vi "Entrada de datos.vi"(5 "ID":string, 6 "string":string) -> (1 "CAN frame":T1 {"payload" format="%x"; "timestamp" format="%<%.7X\n%x>T"; "type" items=["CAN Data"=0, "CAN Remote"=1, "CAN Bus Error"=2, "CAN 2.0 Data"=8, "CAN FD Data"=16, "CAN FD+BRS Data"=24, "J1939 Data"=192, "Delay"=224, "Log Trigger"=225, "Start Trigger"=226]; "identifier" format="%x"})   [LabVIEW 2022 SP3]
uses:
  <vilib>/xnet/xnet.llb/XNET Frame CAN.ctl
  <vilib>/xnet/xnet.llb/XNET Frame Type CAN.ctl
panel:
  out "unsigned byte array":u8[](array[numeric]) format="%x"
  out "number":u32 format="%x"
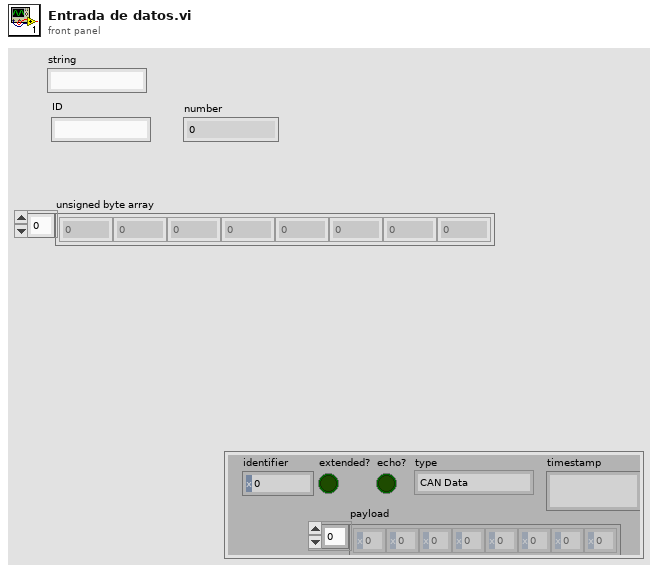
[diagram p1: front panel]
types:
  T1 = typedef "XNET Frame CAN.ctl" = cluster{"timestamp":timestamp, "payload":u8[], "identifier":u32, "type":T2, "extended?":bool, "echo?":bool}
  T2 = typedef "XNET Frame Type CAN.ctl" = u8
  T3 = cluster{"timestamp":timestamp, "unsigned byte array":u8[], u32, "type":T2, "Extended":bool, "Echo":bool}
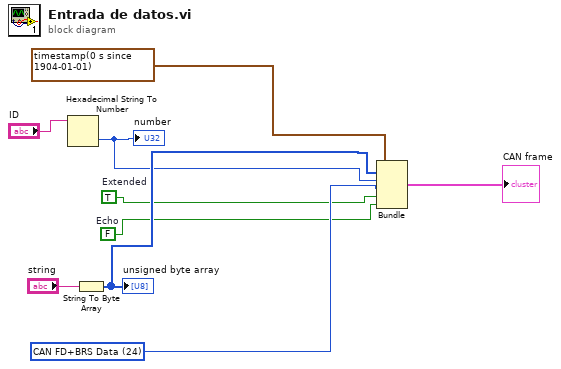
[diagram p0: block diagram]
diagram:
  w4 = T2 24 items=["CAN Data"=0, "CAN Remote"=1, "CAN Bus Error"=2, "CAN 2.0 Data"=8, "CAN FD Data"=16, "CAN FD+BRS Data"=24, "J1939 Data"=192, "Delay"=224, "Log Trigger"=225, "Start Trigger"=226] ("type")
  w2 = FALSE  # Echo
  w3 = TRUE  # Extended
  n1 = Hexadecimal String To Number(string="ID") -> (number=w5:u32)  [unwired: 2 in, 1 out]
  "number" <- w5
  n2 = String To Byte Array(string="string") -> (unsigned byte array=w6:u8[])
  "unsigned byte array" <- w6
  n3 = Bundle("timestamp"=timestamp(0 s since 1904-01-01), "unsigned byte array"=w6, w5, "type"=w4, "Extended"=w3, "Echo"=w2) -> (→"CAN frame":T3)  [unwired: 1 in]
